vi "State_Machine.vi"(8 "error in (no error)":errorcluster caption="entrée d'erreur (pas d'erreur)", 11 "Flash_Jlink en entrée":refnum<class "Nodon_NI_Voltage_Channel_Check.lvclass">) -> (0 "error out":errorcluster caption="sortie d'erreur", 2 "Json_String":string, 3 "Flash_Jlink en sortie":refnum<class "Nodon_NI_Voltage_Channel_Check.lvclass">)   [LabVIEW 2020, in "Library Test.lvlib" / "Nodon_NI_Voltage_Channel_Check.lvclass"]
uses:
  Nodon_NI_Voltage_Channel_Check.lvclass
panel:
  out "String In progress":string
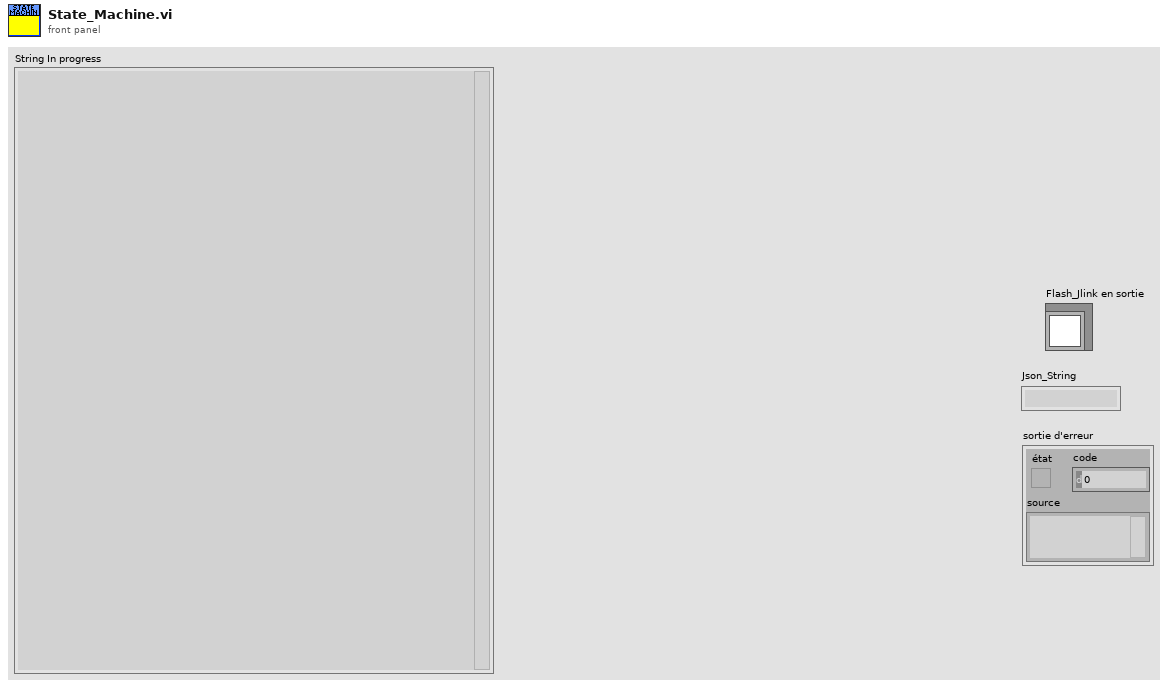
[diagram p1: front panel]
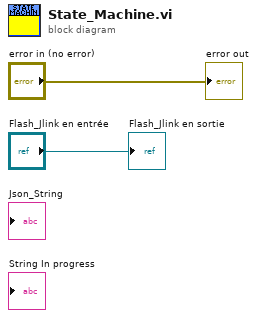
[diagram p0: block diagram]
diagram:
  "Flash_Jlink en sortie" <- "Flash_Jlink en entrée"
  "error out" <- "error in (no error)"
